vi "BCG Lookup.vi"() -> ()   [LabVIEW 2014]
doc: "This example shows how to apply a brightness, contrast, and gamma correction lookup table to an image. These transformations are usually applied to an image to improve its quality as required by a particular application."
uses:
  <vilib>/vision/NI_Vision_Development_Module.lvlib
panel:
  out "Hist-Src":T1(graph)
  out "Image Source":T2(plugin-control)
  out "Dst":T2(plugin-control) caption="Lut Image"
  out "Hist-Dst":T1(graph)
  in  "Stop Button":bool
  in  "BCG":T3={"Brightness"=171.0, "Contrast"=56.0, "Gamma"=2.0} {"Gamma" min=0.1 max=10 step=0.01 scale=10.0..0.1; "Contrast" min=1 max=89 step=1 scale=30.0..60.0; "Brightness" min=0 max=255 step=1 scale=0.0..255.0}
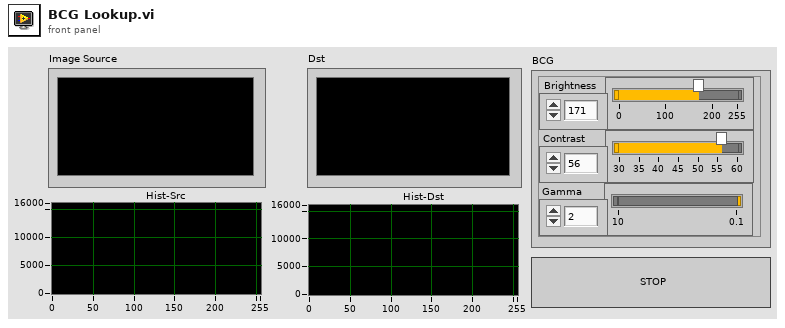
[diagram p1: front panel]
types:
  T1 = cluster{"Starting Value":sgl, "Incremental Value":sgl, "Histogram":u32[]}
  T2 = typedef "IMAQ Image.ctl" = refnum<image>
  T3 = cluster{"Brightness":sgl, "Contrast":sgl, "Gamma":sgl}
  T4 = typedef "Image Type" = u32
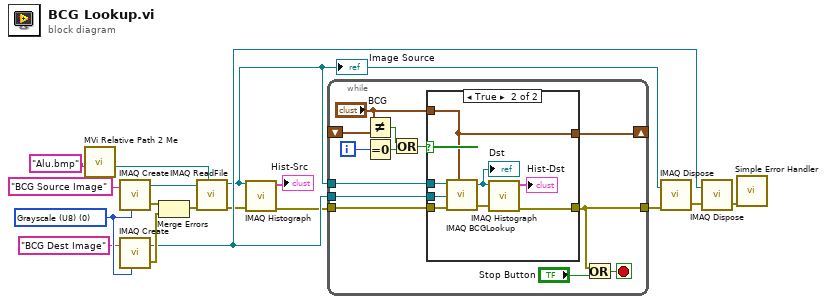
[diagram p0: block diagram]
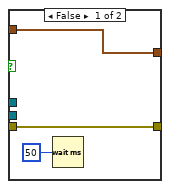
[diagram p2: hidden frame]
diagram:
  w6 = T4 0 items=["Grayscale (U8)", "Grayscale (I16)", "Grayscale (SGL)", "Complex (CSG)", "RGB (U32)", "HSL (U32)", "RGB (U64)", "Grayscale (U16)"] ("Image Type")
  n1 = call "MVi Relative Path 2 Me.vi"("Relative Path"="Alu.bmp" ("name or relative path")) -> ("Appended Dir"=w7:path)  [unwired: 5 in, 1 out]
  n2 = call "IMAQ Create"("Image Name"="BCG Source Image", "Image Type"=w6) -> ("New Image"=w15:T2, "error out"=w14:errorcluster)  [unwired: 3 in]
  n3 = call "IMAQ Create"("Image Name"="BCG Dest Image", "Image Type"=w6) -> ("New Image"=w9:T2, "error out"=w13:errorcluster)  [unwired: 3 in]
  n4 = Merge Errors(w14, w13) -> (w12:errorcluster)
  n5 = call "IMAQ ReadFile"("File Path"=w7, "error in (no error)"=w12, "Image"=w15) -> ("error out"=w4:errorcluster, "Image Out"=w3:T2)  [unwired: 4 in, 3 out]
  "Image Source" <- w3
  n6 = call "IMAQ Histograph"("error in (no error)"=w4, "Image"=w3) -> ("error out"=w2:errorcluster, "Histogram Graph"=→"Hist-Src":T1)  [unwired: 6 in, 2 out]
  n7 = while {
    tunnel: w2 -> [w30]
    tunnel: w3 -> [w29]
    tunnel: w9 -> [w28]
    shift-right: [w27] -> _
    shift-left: _ -> [w26]
    tunnel: [w19] -> w17
    i -> [w24]
    stop <- w18 stop-if-true
    n8 = Not Equal?(x="BCG", y=w26) -> (x != y?=w23:bool)
    n9 = Equal To 0?(x=w24) -> (x = 0?=w22:bool)
    n10 = Or(x=w23, y=w22) -> (x .or. y?=w21:bool)
    n11 = case shown="True" w21 {
      tunnel: w30 -> [w33 w41]
      tunnel: w29 -> [_ w40]
      tunnel: "BCG" -> [w32 w38]
      tunnel: w28 -> [_ w39]
      tunnel: [w32 w38] -> w27
      tunnel: [w33 w36] -> w19
      frame False {
        n12 = Wait (ms)(milliseconds to wait=u32 50) -> ()  [unwired: 1 out]
      }
      frame True {
        n13 = call "IMAQ BCGLookup"("Image Src"=w40, "BCG Values"=w38, "Image Dst"=w39, "error in (no error)"=w41) -> ("Image Dst Out"=w34:T2, "error out"=w37:errorcluster)  [unwired: 3 in]
        "Dst" <- w34
        n14 = call "IMAQ Histograph"("error in (no error)"=w37, "Image"=w34) -> ("error out"=w36:errorcluster, "Histogram Graph"=→"Hist-Dst":T1)  [unwired: 6 in, 2 out]
      }
    }
    n15 = Or(x=w19, y="Stop Button") -> (x .or. y?=w18:bool)
  }
  n16 = call "IMAQ Dispose"("Image"=w3, "error in (no error)"=w17) -> ("error out"=w10:errorcluster)  [unwired: 4 in]
  n17 = call "IMAQ Dispose"("Image"=w9, "error in (no error)"=w10) -> ("error out"=w11:errorcluster)  [unwired: 4 in]
  n18 = call <vilib>:"Simple Error Handler.vi"("error in (no error)"=w11) -> ()  [unwired: 4 in, 5 out]
